vi "Global SETTINGS QH AUTO.vi"() -> ()   [LabVIEW 2019]
panel:
  in  "Fase riscald":enum32{"MANUALE", "AUTO TIMER"}(radio) caption="Fase di riscaldamento"
  in  "Timers":T1
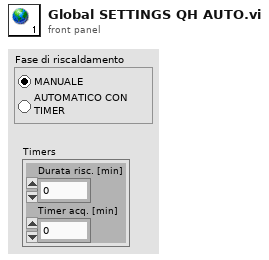
[diagram p1: front panel]
types:
  T1 = cluster{"Durata risc. [min]":dbl, "Timer acq. [min]":dbl}
diagram:
